vi "Index to Cursor Position.vi"(9 "YScale.Ofst&Mult":T2, 10 "XScale.Ofst&Mult":T2, 11 "Index":cluster{"X index":i32, "Y index":i32}) -> (3 "Cursor Position":T1)   [LabVIEW 2016]
uses:
  <vilib>/Utility/miscctls.llb/LVOffsetAndMultiplierTypeDef.ctl
  <vilib>/Utility/miscctls.llb/LVPointDoubleTypeDef.ctl
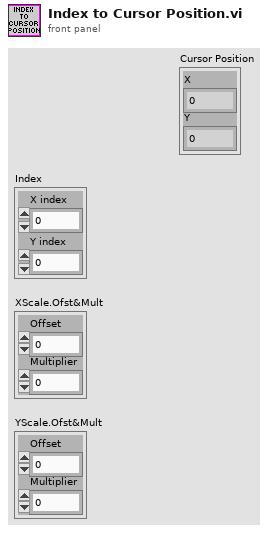
[diagram p1: front panel]
types:
  T1 = typedef "LVPointDoubleTypeDef.ctl" = cluster{"X":dbl, "Y":dbl}
  T2 = typedef "LVOffsetAndMultiplierTypeDef.ctl" = cluster{"Offset":dbl, "Multiplier":dbl}
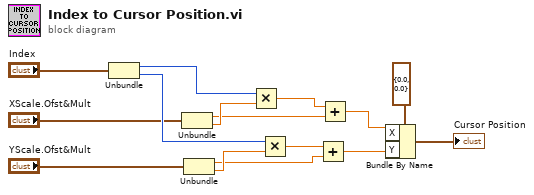
[diagram p0: block diagram]
diagram:
  n1 = Unbundle("Index") -> ("X index"=w8:i32, "Y index"=w7:i32)
  n2 = Unbundle("XScale.Ofst&Mult") -> ("Offset"=w3:dbl, "Multiplier"=w14:dbl)
  n3 = Unbundle("YScale.Ofst&Mult") -> ("Offset"=w1:dbl, "Multiplier"=w13:dbl)
  n4 = Multiply(x=w8, y=w14) -> (x*y=w4:dbl)
  n5 = Multiply(x=w7, y=w13) -> (x*y=w10:dbl)
  n6 = Add(x=w10, y=w1) -> (x+y=w11:dbl)
  n7 = Add(x=w4, y=w3) -> (x+y=w5:dbl)
  n8 = Bundle By Name(cluster=T1 {"X"=0.0, "Y"=0.0} ("Cursor.Cursor Position in"), "X"=w5, "Y"=w11) -> (→"Cursor Position":T1)
